vi "SpecialCannon (SubVI).vi"(10 "Low":dbl[](array[numeric]), 11 "High":bool) -> ()   [LabVIEW 2017]
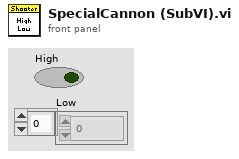
[diagram p1: front panel]
types:
  T1 = typedef "WPI_MotorControlDeviceRef.ctl" = cluster{"DeviceStatus":errorcluster, "Type":T2, "PWM":cluster{"PWM Channel":T3, "DeadBand":T4}, "CAN":cluster{"Device Number":u8, "SetOutput VI Ref":variant, "GetOutput VI Ref":variant, "Enable VI Ref":variant, "Disable VI Ref":variant, "Data":variant}, "Invert":bool, "DIO PWM":cluster{"PWM \"Enable\" Channel":T3, "DIOChannel":T5, "PWM Rate":dbl}}
  T2 = typedef "WPI_MotorControlType.ctl" = enum16{"PWM", "CAN", "DIO PWM"}
  T3 = typedef "FPGA_DIOPWMChannel.ctl" = enum8{"PWM 0", "PWM 1", "PWM 2", "PWM 3", "PWM 4", "PWM 5", "PWM 6", "PWM 7", "PWM 8", "PWM 9", "PWM MXP 0", "PWM MXP 1", "PWM MXP 2", "PWM MXP 3", "PWM MXP 4", "PWM MXP 5", "PWM MXP 6", "PWM MXP 7", "PWM MXP 8", "PWM MXP 9", "Invalid"}
  T4 = typedef "WPI_PWMDeadband.ctl" = cluster{"Name":string, "maxPositivePwm":i32, "minPositivePwm":i32, "centerPwm":i32, "maxNegativePwm":i32, "minNegativePwm":i32, "angularRange":u16}
  T5 = typedef "FPGA_DIOChannel.ctl" = enum8{"DIO 0", "DIO 1", "DIO 2", "DIO 3", "DIO 4", "DIO 5", "DIO 6", "DIO 7", "DIO 8", "DIO 9", "DIO MXP 0", "DIO MXP 1", "DIO MXP 2", "DIO MXP 3", "DIO MXP 4", "DIO MXP 5", "DIO MXP 6", "DIO MXP 7", "DIO MXP 8", "DIO MXP 9", "DIO MXP 10", "DIO MXP 11", "DIO MXP 12", "DIO MXP 13", "DIO MXP 14", "DIO MXP 15", "SPI Port CS1", "SPI Port CS2", "SPI Port CS3", "SPI Port MISO", "SPI Port MOSI", "Invalid"}
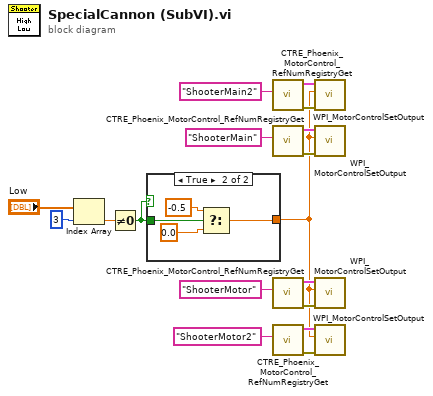
[diagram p0: block diagram]
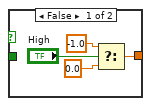
[diagram p2: hidden frame]
diagram:
  n1 = Index Array(array="Low", index=3) -> (element=w4:dbl)
  n2 = Not Equal To 0?(x=w4) -> (x != 0?=w3:bool)
  n3 = case shown="True" w3 {
    tunnel: w3 -> [_ w25]
    tunnel: [w18 w22] -> w2
    frame False {
      n4 = Select(t=-1.0, s="High", f=0.0) -> (s? t:f=w18:dbl)
    }
    frame True {
      n5 = Select(t=-0.5, s=w25, f=0.0) -> (s? t:f=w22:dbl)
    }
  }
  n6 = call "CTRE_Phoenix_MotorControl_RefNumRegistryGet.vi"("refnum name"="ShooterMain2") -> ("error out"=w14:errorcluster, "PhoenixMotorControlDevRef"=w13:T1)  [unwired: 9 in]
  n7 = call "CTRE_Phoenix_MotorControl_RefNumRegistryGet.vi"("refnum name"="ShooterMain") -> ("error out"=w11:errorcluster, "PhoenixMotorControlDevRef"=w12:T1)  [unwired: 9 in]
  n8 = call "CTRE_Phoenix_MotorControl_RefNumRegistryGet.vi"("refnum name"="ShooterMotor") -> ("error out"=w16:errorcluster, "PhoenixMotorControlDevRef"=w15:T1)  [unwired: 9 in]
  n9 = call "CTRE_Phoenix_MotorControl_RefNumRegistryGet.vi"("refnum name"="ShooterMotor2") -> ("error out"=w1:errorcluster, "PhoenixMotorControlDevRef"=w17:T1)  [unwired: 9 in]
  n10 = call <vilib>:"WPI_MotorControlSetOutput.vi"("error in (no error)"=w14, "Output"=w2, "MotorControlDevRef"=w13) -> ()  [unwired: 6 in, 3 out]
  n11 = call <vilib>:"WPI_MotorControlSetOutput.vi"("error in (no error)"=w11, "Output"=w2, "MotorControlDevRef"=w12) -> ()  [unwired: 6 in, 3 out]
  n12 = call <vilib>:"WPI_MotorControlSetOutput.vi"("error in (no error)"=w16, "Output"=w2, "MotorControlDevRef"=w15) -> ()  [unwired: 6 in, 3 out]
  n13 = call <vilib>:"WPI_MotorControlSetOutput.vi"("error in (no error)"=w1, "Output"=w2, "MotorControlDevRef"=w17) -> ()  [unwired: 6 in, 3 out]
